vi "PDLM_GetLaserMode.vi"(8 "error in (no error)":errorcluster, 11 "USBIdx":i32) -> (0 "error out":errorcluster, 2 "mode":T1, 3 "return type":i32)   [LabVIEW 2017]
uses:
  PDLM_LaserMode.ctl
  PDLM_DllPath_global.vi
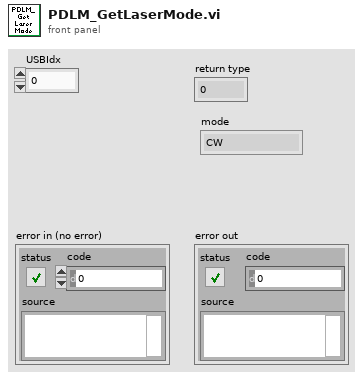
[diagram p1: front panel]
types:
  T1 = typedef "PDLM_LaserMode.ctl" = enum32{"CW", "PULSE", "BURST"}
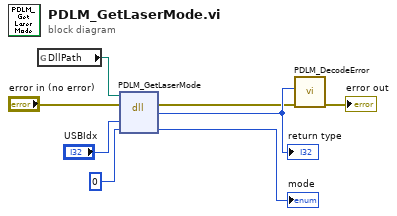
[diagram p0: block diagram]
diagram:
  n1 = global read "PDLM_DllPath_global.vi" "DllPath"() -> (w4:path)
  n2 = dll-call lib="M:/_dev/progs/LabVIEW/_lib/PQ/Taiko/pdlm_lib.dll" fn="PDLM_GetLaserMode"(path in=w4, error in="error in (no error)", "USBIdx"="USBIdx", "mode"=u32 0) -> (error out=w6:errorcluster, "return type"=w7:i32, "mode"=→"mode":u32)  [unwired: 2 in, 1 out]
  "return type" <- w7
  n3 = call "PDLM_DecodeError.vi"("error in (no error)"=w6, "code"=w7) -> ("error out"=→"error out":errorcluster)  [unwired: 7 in, 2 out]
